vi "Cleanup.vi"(8 "error in (no error)":errorcluster, 11 "SolutionBuilder in":refnum<class "SolutionBuilder.lvclass">) -> (0 "error out":errorcluster, 3 "SolutionBuilder out":refnum<class "SolutionBuilder.lvclass">)   [LabVIEW 2020, in "SolutionBuilder.lvlib" / "SolutionBuilder.lvclass"]
uses:
  SolutionBuilder.lvclass
  Private/FileInfo.ctl
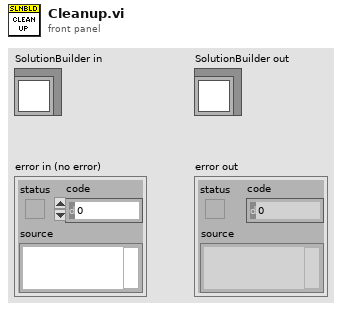
[diagram p1: front panel]
types:
  T1 = typedef "SolutionBuilder.lvlib/SolutionBuilder.lvclass/FileInfo.ctl" = cluster{"Library ref":refnum<vi>, "Target path":path, "Source name":string, "Build spec name":string}
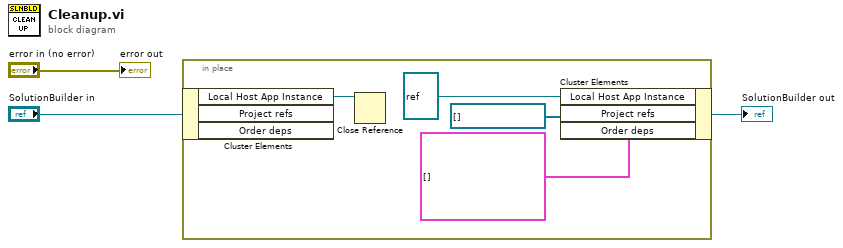
[diagram p0: block diagram]
diagram:
  n1 = in-place {
    n2 = in-place-cluster #1("SolutionBuilder in") -> ("Local Host App Instance"=w7:refnum<vi>)  [unwired: 2 out]
    n3 = Close Reference(reference=w7) -> ()  [unwired: 1 in, 1 out]
    n4 = in-place-cluster #1("Local Host App Instance"=refnum<vi> refnum, "Project refs"=refnum<vi>[] [], "Order deps"=T1[] []) -> (→"SolutionBuilder out":refnum<class "SolutionBuilder.lvclass">)
  }
  "error out" <- "error in (no error)"
